vi "UnloadAction.vi"(8 "error in (no error)":errorcluster caption="entrée d'erreur (pas d'erreur)", 11 "Tools In":refnum<class "BNC845.lvclass"> caption="DNL_LabVIEW Object in") -> (0 "error out":errorcluster caption="sortie d'erreur", 3 "Tools Out":refnum<class "BNC845.lvclass"> caption="DNL_LabVIEW Object out")   [LabVIEW 2019, in "BNC845.lvclass"]
uses:
  BNC845.lvclass
  C:/Programmes Labview/LabScanV1A/DevicesClass/BaseDevice/BaseDevice.lvclass
  BaseDevice/BaseDevice.lvclass
  <instrlib>/Berkeley Nucleonics 845/Berkeley Nucleonics 845.lvlib
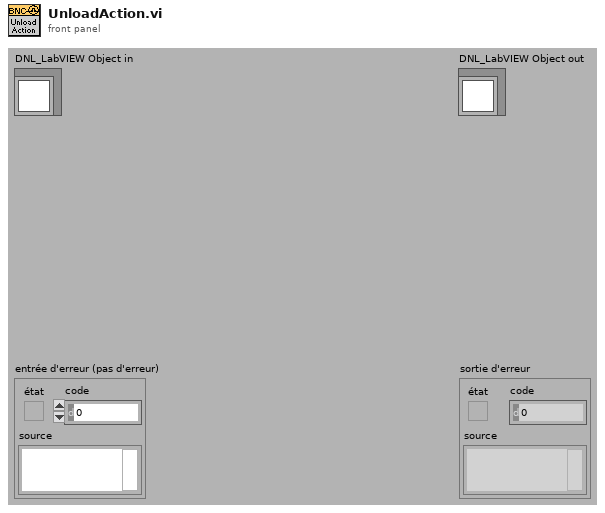
[diagram p1: front panel]
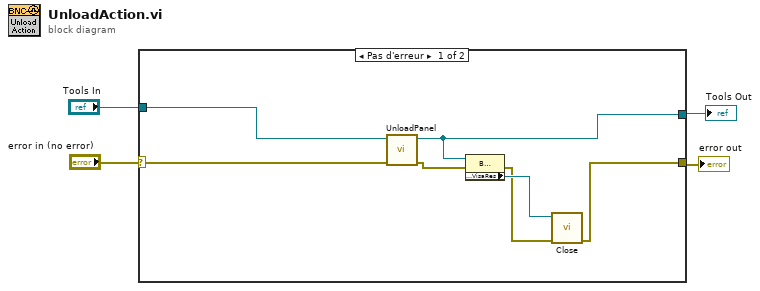
[diagram p0: block diagram]
diagram:
  n1 = case shown="Pas d'erreur" "error in (no error)" {
    selector: "error in (no error)" -> [w11 w12]
    tunnel: [w5 w12] -> w3
    tunnel: [w9 w13] -> w2
    tunnel: "Tools In" -> [w10 w13]
    frame No Error {
      n2 = call "UnloadPanel.vi"("error in (no error)"=w11, "Device en entrée"=w10) -> ("error out"=w8:errorcluster, "Device en sortie"=w9:refnum<class "BNC845.lvclass">)  [unwired: 8 in]
      n3 = property class="BNC845.lvclass"(reference=w9, error in=w8) -> (error out=w6:errorcluster, "Accessor:VisaRes"=w7:refnum<visa-resource-name>)  [unwired: 1 out]
      n4 = call <instrlib>:"Close.vi"("error in (no error)"=w6, "VISA resource name"=w7) -> ("error out"=w5:errorcluster)  [unwired: 9 in]
    }
    frame Error {
    }
  }
  "error out" <- w3
  "Tools Out" <- w2
